vi "Configure Record Data (Display).vi"(0 "VISA resource name":refnum<visa-resource-name>, 5 "Record Number (1)":i32=1 min=1 max=440 step=1, 7 "Kind of Channel (0: Off)":u16(ring) items=["Off", "IO", "Math", "Com"], 9 "Channel Number (0001)":string="0001", 11 "error in (no error)":errorcluster) -> (4 "VISA resource name out":refnum<visa-resource-name>, 6 "Record Number":i32, 15 "error out":errorcluster)   [LabVIEW 2020, in "Yokogawa GX Series.lvlib"]
doc: "Sets channel for recording display data.\n\nCommand: SRecDisp"
uses:
  <instrlib>/Yokogawa GX Series/Yokogawa GX Series.lvlib
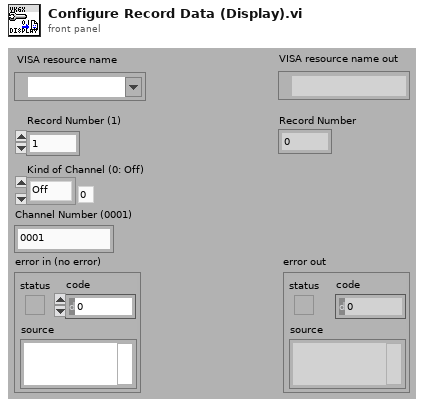
[diagram p1: front panel]
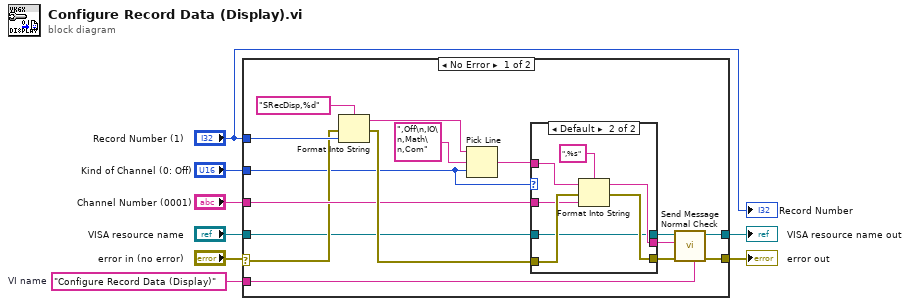
[diagram p0: block diagram]
diagram:
  w8 = "Configure Record Data (Display)"  # VI name
  n1 = case shown="No Error" "error in (no error)" {
    selector: "error in (no error)" -> [w13 w35]
    tunnel: w8 -> [w24 _]
    tunnel: "VISA resource name" -> [w10 w36]
    tunnel: [w23 w36] -> w6
    tunnel: [w22 w35] -> w5
    tunnel: "Kind of Channel (0: Off)" -> [w11 _]
    tunnel: "Record Number (1)" -> [w20 _]
    tunnel: "Channel Number (0001)" -> [w16 _]
    frame No Error {
      n2 = Format Into String(format string="SRecDisp,%d", error in=w13, w20) -> (resulting string=w21:string, error out=w17:errorcluster)  [unwired: 1 in]
      n3 = Pick Line(string ("")=w21, multi-line string=",Off\n,IO\n,Math\n,Com", line index=w11) -> (output string=w18:string)
      n4 = case shown="Default" w11 {
        tunnel: w18 -> [w25 w34]
        tunnel: w17 -> [w26 w32]
        tunnel: w16 -> [_ w31]
        tunnel: [w26 w30] -> w15
        tunnel: [w25 w29] -> w14
        tunnel: w10 -> [w27 w28]
        tunnel: [w27 w28] -> w9
        frame 0 {
        }
        frame Default {
          n5 = Format Into String(format string=",%s", initial string=w34, error in=w32, w31) -> (resulting string=w29:string, error out=w30:errorcluster)
        }
      }
      n6 = call <instrlib>:"Send Message Normal Check.vi"("Source (\"\")"=w24, "error in (no error)"=w15, "Send Message (\"\")"=w14, "VISA resource name"=w9) -> ("error out"=w22:errorcluster, "VISA resource name out"=w23:refnum<visa-resource-name>)  [unwired: 1 in, 5 out]
    }
    frame Error {
    }
  }
  "error out" <- w5
  "VISA resource name out" <- w6
  "Record Number" <- "Record Number (1)"
